vi "BrowseRecipe.vi"(8 "error in (no error)":errorcluster) -> (0 "error out":errorcluster, 2 "cancelled":bool, 3 "selected path":path)   [LabVIEW 2019]
uses:
  <vilib>/Utility/sysdir.llb/System Directory Type.ctl
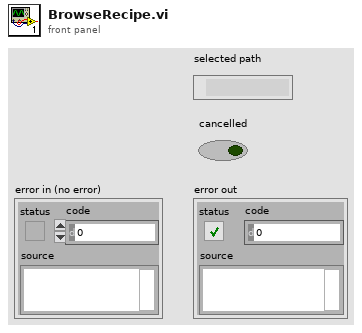
[diagram p1: front panel]
types:
  T1 = typedef "System Directory Type.ctl" = i32
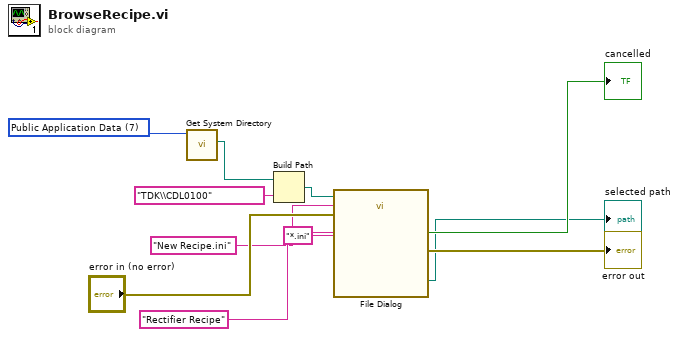
[diagram p0: block diagram]
diagram:
  w1 = T1 7 items=["User Home"=0, "User Desktop"=1, "User Documents"=2, "User Application Data"=3, "User Preferences"=4, "User Temporary"=5, "Public Documents"=6, "Public Application Data"=7, "Public Preferences"=8, "Public Cache"=13, "System Core Libraries"=9, "System Installed Libraries"=10, "Application Files"=11, "Boot Volume Root"=12] ("system directory type")
  n1 = call <vilib>:"Get System Directory.vi"("system directory type"=w1) -> ("system directory"=w2:path)  [unwired: 10 in]
  n2 = Build Path(base path=w2, name or relative path="TDK\\CDL0100") -> (appended path=w4:path)
  n3 = call "File Dialog"("start path"=w4, "default name"="New Recipe.ini", "error in"="error in (no error)", "pattern (all files)"="*.ini", "pattern label"="Rectifier Recipe") -> ("selected path"=→"selected path":path, "cancelled"=→"cancelled":bool, "error out"=→"error out":errorcluster)  [unwired: 7 in, 1 out]
